vi "TTL high-low control.vi"(8 "error in":errorcluster, 9 "TTL outputs":bool[](array[boolean]), 10 "Channels":string[](array[string]), 11 "Handle in":i32) -> (0 "error out":errorcluster, 3 "Handle out":i32)   [LabVIEW 2018]
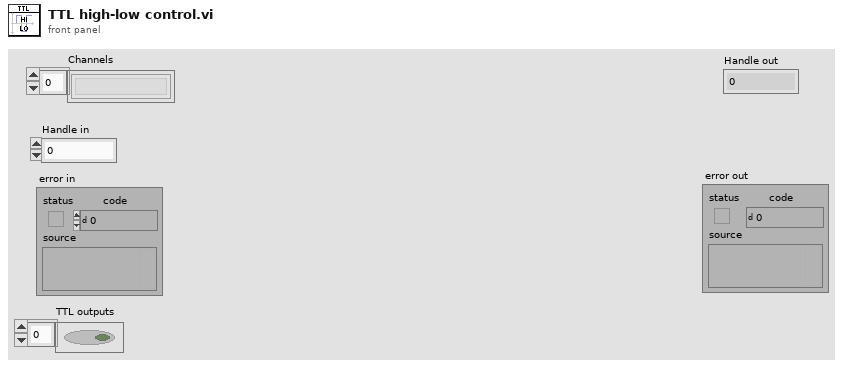
[diagram p1: front panel]
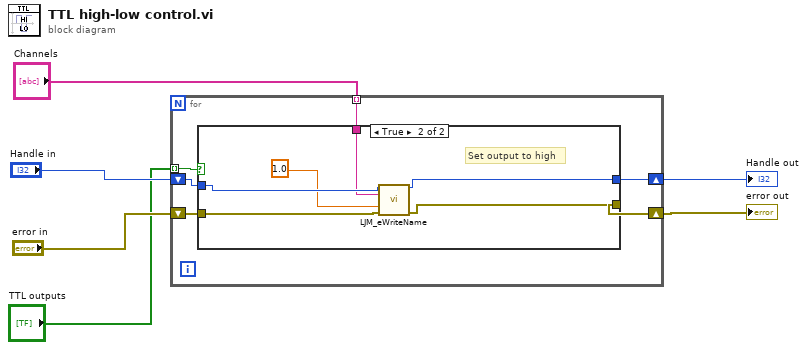
[diagram p0: block diagram]
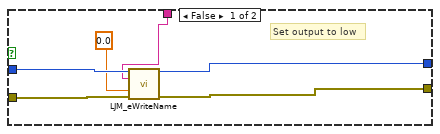
[diagram p2: hidden frame]
diagram:
  n1 = for {
    tunnel: "Channels" -> [w12] mode=indexing
    shift-right: [w9] -> w3
    shift-left: "Handle in" -> [w11]
    shift-right: [w8] -> w2
    shift-left: "error in" -> [w10]
    tunnel: "TTL outputs" -> [w7] mode=indexing
    n2 = case shown="True" w7 {
      tunnel: w11 -> [w18 w24]
      tunnel: [w14 w21] -> w8
      tunnel: w10 -> [w17 w22]
      tunnel: [w15 w20] -> w9
      tunnel: w12 -> [w13 w23]
      frame False {
        # "Set output to low"
        n3 = call "LJM_eWriteName.vi"("Handle In"=w18, "Name"=w13, "Value"=0.0, "error in"=w17) -> ("Handle Out"=w15:i32, "error out"=w14:errorcluster)  [unwired: 10 in]
      }
      frame True {
        # "Set output to high"
        n4 = call "LJM_eWriteName.vi"("Handle In"=w24, "Name"=w23, "Value"=1.0, "error in"=w22) -> ("Handle Out"=w20:i32, "error out"=w21:errorcluster)  [unwired: 10 in]
      }
    }
  }
  "Handle out" <- w3
  "error out" <- w2
